vi "url2filen.vi"(6 "srcurl":string) -> (1 "virtual path":string)   [LabVIEW 2010]
uses:
  <vilib>/addons/internet/NI_InternetTK_Core_VIs.lvlib
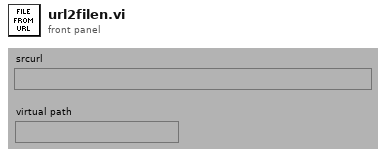
[diagram p1: front panel]
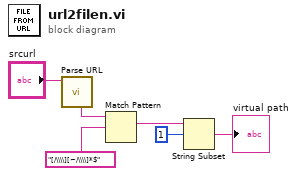
[diagram p0: block diagram]
diagram:
  n1 = call <vilib>:"Parse URL.vi"("URL"="srcurl") -> ("virtual path"=w1:string)  [unwired: 5 in, 5 out]
  n2 = Match Pattern(string=w1, regular expression="[/\\\\][~/\\\\]*$") -> (match substring=w5:string)  [unwired: 4 out]
  n3 = String Subset(string=w5, offset (0)=1) -> (substring=→"virtual path":string)  [unwired: 1 in]
